vi "removeEdge.vi"(0 "reference":refnum<class "AbstractNode.lvclass">, 1 "graph":refnum<class "Graph.lvclass">, 2 "edge":refnum<class "AbstractEdge.lvclass">, 5 "error in (no error)":errorcluster) -> (14 "reference out":refnum<class "AbstractNode.lvclass">, 19 "error out":errorcluster)   [LabVIEW 2016, in "AbstractNode.lvclass"]
uses:
  <resource>/Framework/Providers/Open_GDS/UML/AbstractNode_class/AbstractNode.lvclass
  <resource>/Framework/Providers/Open_GDS/UML/Graph_class/Graph.lvclass
  <resource>/Framework/Providers/Open_GDS/UML/AbstractEdge_class/AbstractEdge.lvclass
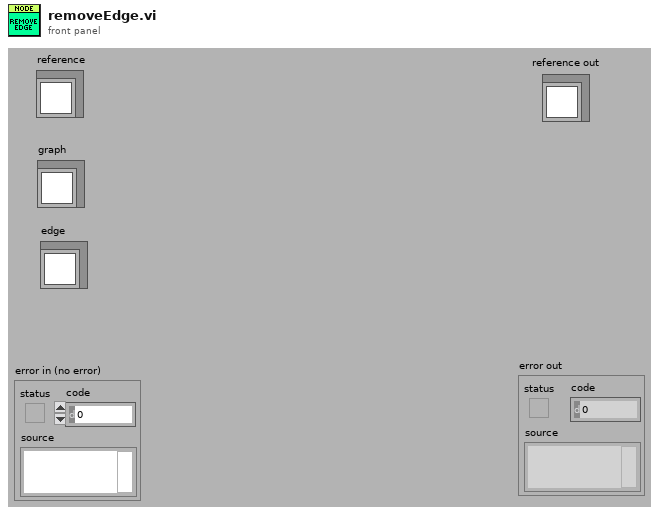
[diagram p1: front panel]
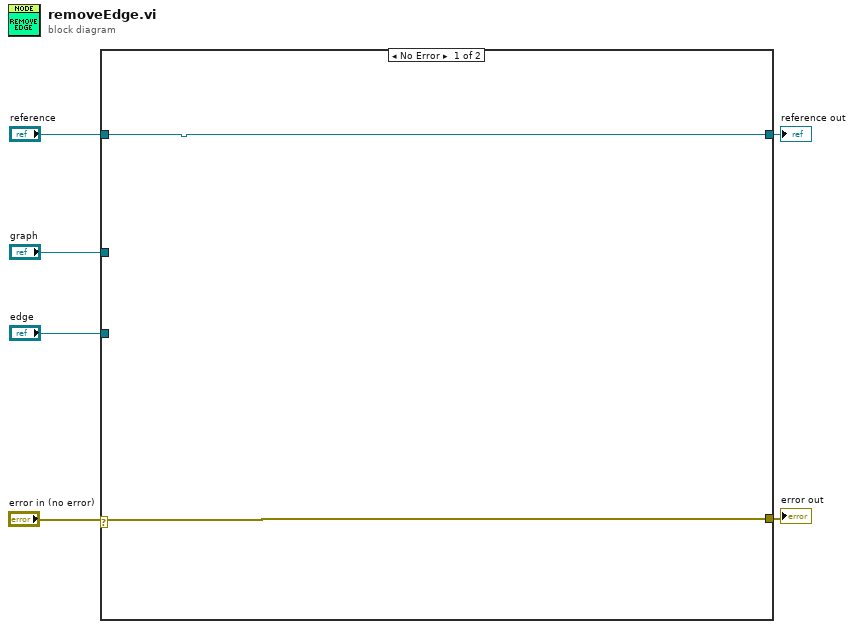
[diagram p0: block diagram]
diagram:
  n1 = case shown="No Error" "error in (no error)" {
    selector: "error in (no error)" -> [w7 w9]
    tunnel: "reference" -> [w8 w10]
    tunnel: [w7 w9] -> w5
    tunnel: [w8 w10] -> w4
    tunnel: "graph" -> [_ _]
    tunnel: "edge" -> [_ _]
    frame No Error {
    }
    frame Error {
    }
  }
  "reference out" <- w4
  "error out" <- w5
